vi "Pcre2SubstringLengthByName8.vi"(8 "error in":errorcluster, 10 "Name":string, 11 "pMatchData":u64 format="%.0x") -> (0 "error out":errorcluster, 1 "Length":u64, 3 "pMatchData":u64 format="%.0x")   [LabVIEW 2021, in "libpcre2-8.lvlib"]
uses:
  libpcre2-8.lvlib
  libpcre2-8-x32.dll
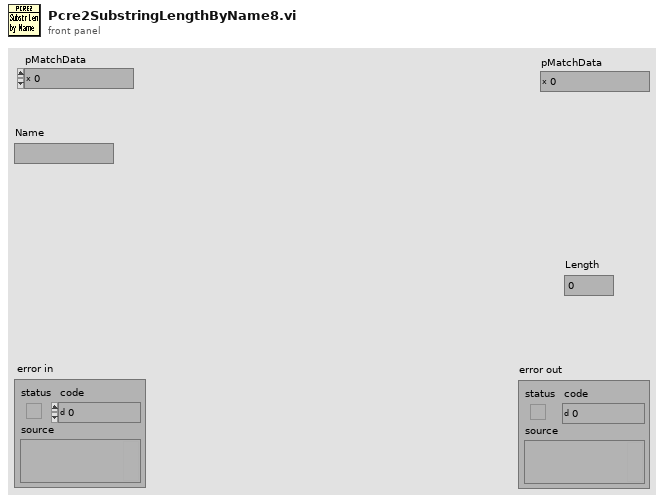
[diagram p1: front panel]
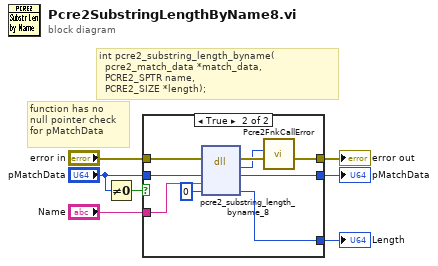
[diagram p0: block diagram]
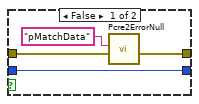
[diagram p2: hidden frame]
diagram:
  # "function has no \nnull pointer check \nfor pMatchData"
  # "int pcre2_substring_length_byname(\n  pcre2_match_data *match_data, \n  PCRE2_SPTR name, \n  PCRE2_SIZE *length);"
  n1 = Not Equal To 0?(x="pMatchData") -> (x != 0?=w3:bool)
  n2 = case shown="True" w3 {
    tunnel: "error in" -> [w10 w20]
    tunnel: [w9 w15] -> w6
    tunnel: "pMatchData" -> [w11 w19]
    tunnel: [w11 w18] -> w5
    tunnel: [_ w17] -> w4
    tunnel: "Name" -> [_ w13]
    frame False {
      n3 = call "Pcre2ErrorNull.vi"("error in"=w10, "What"="pMatchData" ("message")) -> ("error out"=w9:errorcluster)  [unwired: 9 in]
    }
    frame True {
      n4 = dll-call lib="libpcre2-8-x*.dll" fn="pcre2_substring_length_byname_8"(error in=w20, "match_data"=w19, "name"=w13, "length"=u64 0) -> (error out=w16:errorcluster, "return type"=w14:i32, "match_data"=w18:u64, "length"=w17:u64)  [unwired: 3 in, 1 out]
      n5 = call "Pcre2FnkCallError.vi"("error in"=w16, "ErrorCode"=w14) -> ("error out"=w15:errorcluster)  [unwired: 9 in]
    }
  }
  "pMatchData" <- w5
  "error out" <- w6
  "Length" <- w4
